vi "interfejs.vi"(11 "wejście":errorcluster) -> ()   [LabVIEW 2014]
uses:
  glownaMaszynaStanowVIs/wczytajListePunktowVIs/RodzajPomiarow.ctl
  glownaMaszynaStanowVIs/AkcjaGFV.ctl
panel:
  in  "Wybierz rodzaj pomiarów:":T1
  out "Zrealizowane punkty:":string
  in  "Nadawcza/odbiorcza":bool
  out "Odb. góra":bool
  out "Odb. dół":bool
  out "Odb. prawo":bool
  out "Odb. lewo":bool
  out "Pomiar":bool
  in  "Stop":bool
  in  "Dӣ":bool
  in  "GÓRA":bool
  in  "LEWO":bool
  in  "PRAWO":bool
  in  "Włącz/wyłącz":bool
  in  "Start":bool
  out "Działanie ramienia":bool
  out "Nad. góra":bool
  out "Nad. dół":bool
  out "Nad. prawo":bool
  out "Nad. lewo":bool
  # "Komora nadawcza"
  # "Praca ręczna"
  # "Komora odbiorcza"
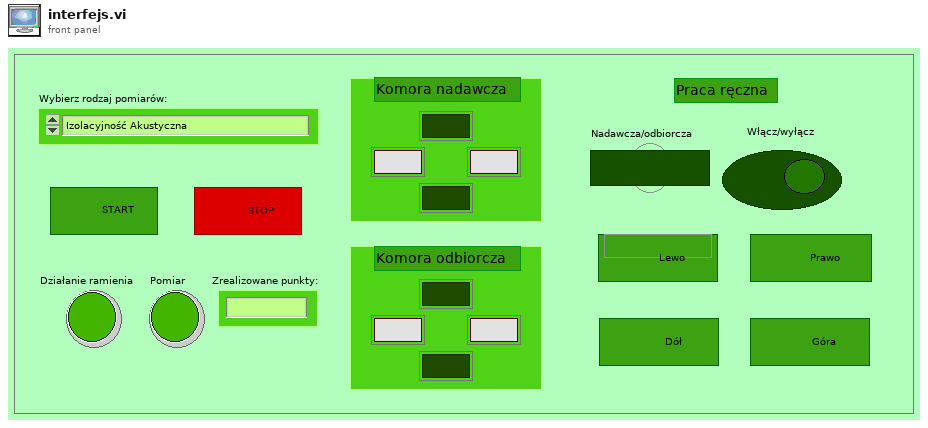
[diagram p1: front panel]
types:
  T1 = typedef "RodzajPomiarow.ctl" = enum16{"Izolacyjność Akustyczna"}
  T2 = typedef "WyjsciaParametry.ctl" = cluster{"Nad. lewo":bool, "Nad.  prawo":bool, "Nad.  góra":bool, "Nad. dół":bool, "Działanie":bool, "Pomiar":bool, "Odb. dół":bool, "Odb.  góra":bool, "Odb.  prawo":bool, "Odb. lewo":bool, "Punkty pom. info":string}
  T3 = typedef "WejsciaParametry.ctl" = cluster{"LEWO":bool, "PRAWO":bool, "GÓRA":bool, "Dӣ":bool, "Stop":bool, "Start":bool, "Praca ręczna":bool, "Komora":bool, "Rodzaj pomiarów":T1}
  T4 = typedef "AkcjaGFV.ctl" = enum16{"Czytaj", "Zapisz", "Reset"}
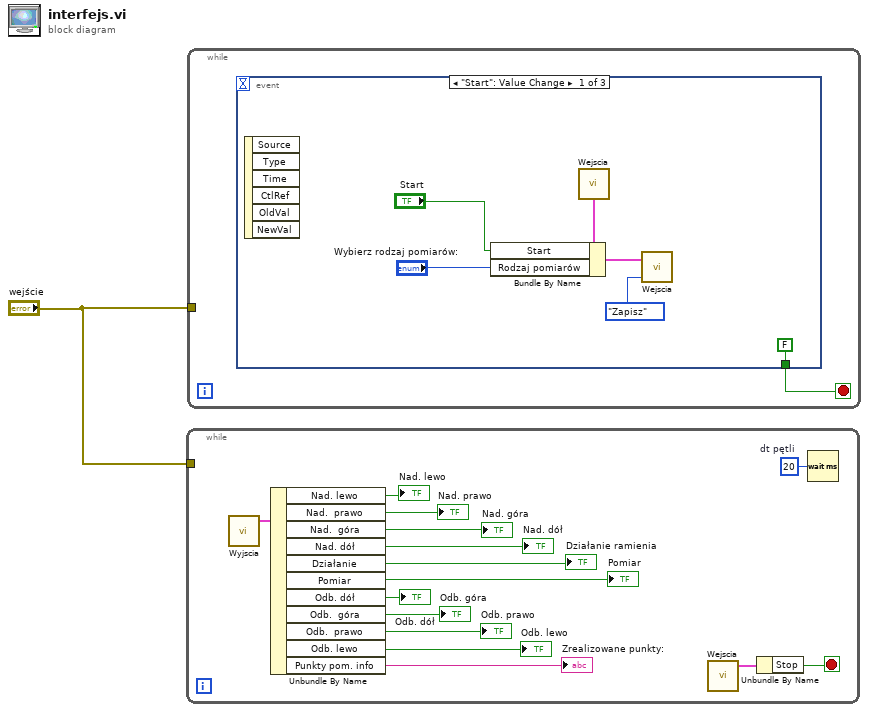
[diagram p0: block diagram]
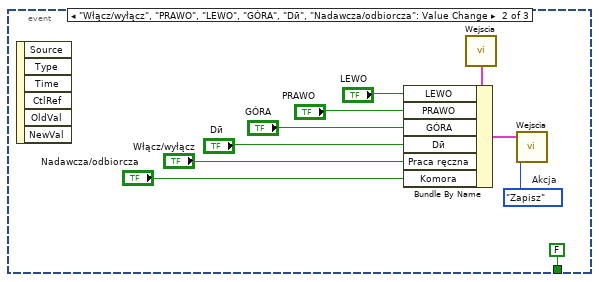
[diagram p2: hidden frame]
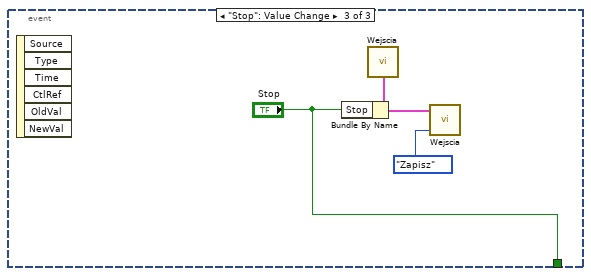
[diagram p3: hidden frame]
diagram:
  n1 = while {
    tunnel: "wejście" -> [_]
    stop <- w8 stop-if-true
    w16 = u32 20  # dt pętli
    n2 = call "Wyjscia.vi"() -> ("Wyjście"=w15:T2)  [unwired: 5 in]
    n3 = Unbundle By Name(w15) -> ("Nad. lewo"=→"Nad. lewo":bool, "Nad.  prawo"=→"Nad. prawo":bool, "Nad.  góra"=→"Nad. góra":bool, "Nad. dół"=→"Nad. dół":bool, "Działanie"=→"Działanie ramienia":bool, "Pomiar"=→"Pomiar":bool, "Odb. dół"=→"Odb. dół":bool, "Odb.  góra"=→"Odb. góra":bool, "Odb.  prawo"=→"Odb. prawo":bool, "Odb. lewo"=→"Odb. lewo":bool, "Punkty pom. info"=→"Zrealizowane punkty:":string)
    n4 = call "Wejscia.vi"() -> ("Wyjście"=w9:T3)  [unwired: 5 in]
    n5 = Unbundle By Name(w9) -> ("Stop"=w8:bool)
    n6 = Wait (ms)(milliseconds to wait=w16) -> ()  [unwired: 1 out]
  }
  n7 = while {
    tunnel: "wejście" -> [_]
    stop <- w17 stop-if-true
    n8 = event shown="[0] \"Start\": Value Change" {
      selector: _ -> [_ _ _]
      dyn-events: _ -> [_ _ _]
      timeout: _ -> [_ _ _]
      tunnel: [FALSE ("Stop") FALSE ("Stop") "Stop"] -> w17
      event "Start": Value Change {
        n9 = event-data() -> ()  [unwired: 1 in, 6 out]
        n10 = call "Wejscia.vi"() -> ("Wyjście"=w21:T3)  [unwired: 5 in]
        n11 = Bundle By Name(cluster=w21, "Start"="Start", "Rodzaj pomiarów"="Wybierz rodzaj pomiarów:") -> (w23:T3)
        n12 = call "Wejscia.vi"("Akcja"=AkcjaGFV."Zapisz", "Wejście"=w23) -> ()  [unwired: 3 in, 1 out]
      }
      event "Włącz/wyłącz", "PRAWO", "LEWO", "GÓRA", "Dӣ", "Nadawcza/odbiorcza": Value Change {
        w31 = AkcjaGFV."Zapisz"  # Akcja
        n13 = event-data() -> ()  [unwired: 1 in, 6 out]
        n14 = call "Wejscia.vi"() -> ("Wyjście"=w25:T3)  [unwired: 5 in]
        n15 = Bundle By Name(cluster=w25, "LEWO"="LEWO", "PRAWO"="PRAWO", "GÓRA"="GÓRA", "Dӣ"="Dӣ", "Praca ręczna"="Włącz/wyłącz", "Komora"="Nadawcza/odbiorcza") -> (w30:T3)
        n16 = call "Wejscia.vi"("Akcja"=w31, "Wejście"=w30) -> ()  [unwired: 3 in, 1 out]
      }
      event "Stop": Value Change {
        n17 = event-data() -> ()  [unwired: 1 in, 6 out]
        n18 = call "Wejscia.vi"() -> ("Wyjście"=w35:T3)  [unwired: 5 in]
        n19 = Bundle By Name(cluster=w35, "Stop"="Stop") -> (w37:T3)
        n20 = call "Wejscia.vi"("Akcja"=AkcjaGFV."Zapisz", "Wejście"=w37) -> ()  [unwired: 3 in, 1 out]
      }
    }
  }
